vi "Generate RPC Messages.vi"(6 "Enum Metadata":T4[](array[typedef]), 7 "Messages Metadata":T5[](array[typedef]), 8 "error in (no error)":errorcluster, 11 "Library":refnum<vi>) -> (0 "error out":errorcluster, 3 "Library":refnum<vi>)   [LabVIEW 2019, in "gRPC Template Creation Utility.lvlib"]
uses:
  gRPC Template Creation Utility.lvlib
  TypeDefs/Message Metadata (Scripting).ctl
  TypeDefs/Message Element Metadata (Scripting).ctl
  TypeDefs/Message Element Type.ctl
  TypeDefs/Enum Metadata (Scripting).ctl
  TypeDefs/Oneof Metadata.ctl
panel:
  in  "Oneof Metadata":T1[](array[typedef])
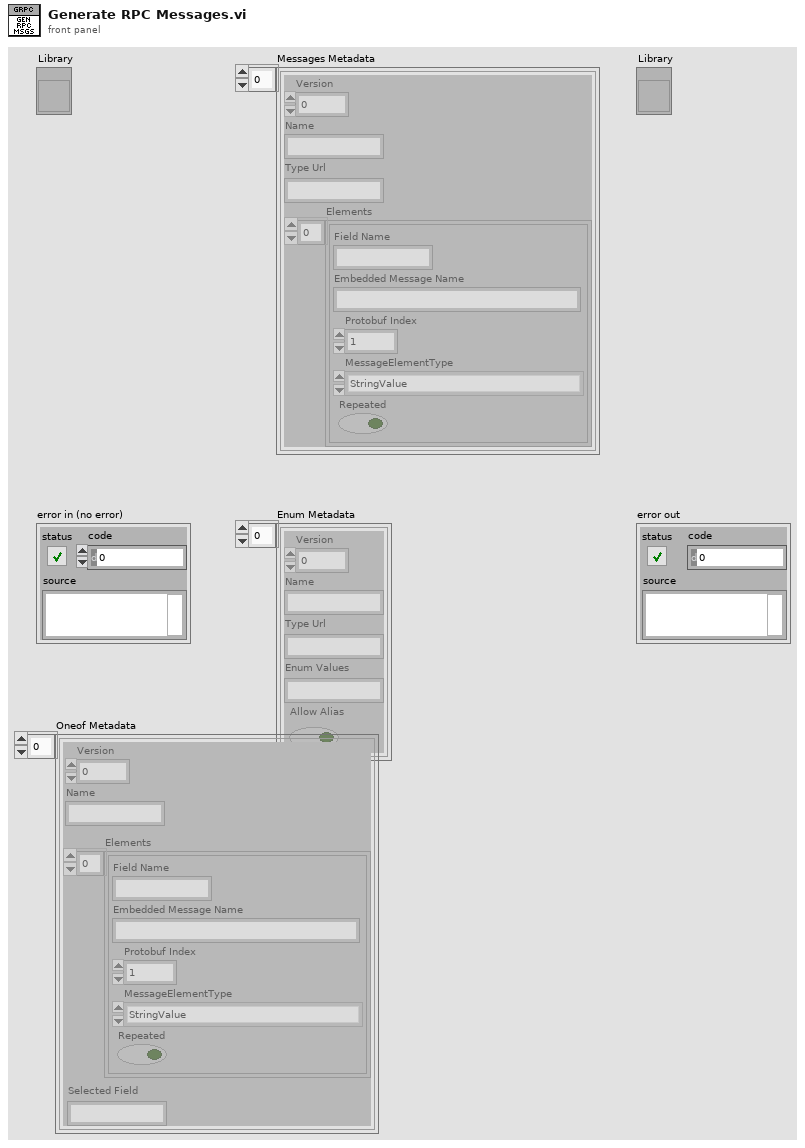
[diagram p1: front panel]
types:
  T1 = typedef "gRPC Template Creation Utility.lvlib/Oneof Metadata.ctl" = cluster{"Version":i32, "Name":string, "Elements":T2[], "Selected Field":string}
  T2 = typedef "gRPC Template Creation Utility.lvlib/Message Element Metadata (Scripting).ctl" = cluster{"Field Name":string, "Embedded Message Name":string, "Protobuf Index":i32, "MessageElementType":T3, "Repeated":bool}
  T3 = typedef "gRPC Template Creation Utility.lvlib/Message Element Type.ctl" = enum32{"Int32Value", "FloatValue", "DoubleValue", "BoolValue", "StringValue", "MessageValue", "Int64Value", "UInt32Value", "UInt64Value", "EnumValue", "Bytes", "Fixed64", "Fixed32", "SFixed64", "SFixed32", "SInt64", "SInt32", "Oneof"}
  T4 = typedef "gRPC Template Creation Utility.lvlib/Enum Metadata (Scripting).ctl" = cluster{"Version":i32, "Name":string, "Type Url":string, "Enum Values":string, "Allow Alias":bool}
  T5 = typedef "gRPC Template Creation Utility.lvlib/Message Metadata (Scripting).ctl" = cluster{"Version":i32, "Name":string, "Type Url":string, "Elements":T2[]}
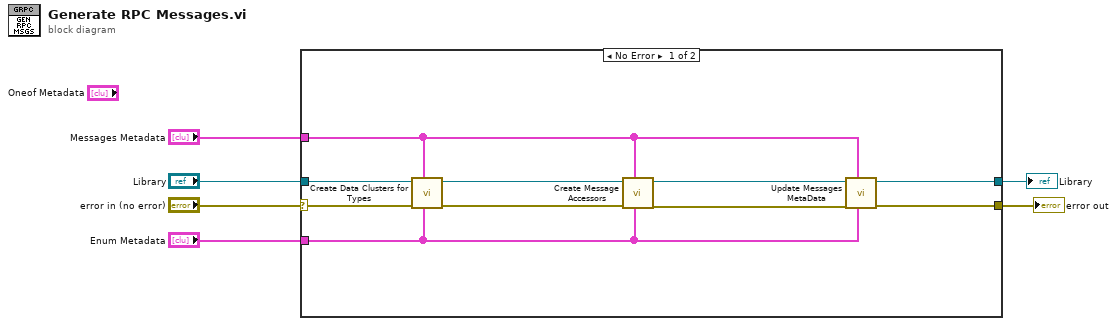
[diagram p0: block diagram]
diagram:
  n1 = case shown="No Error" "error in (no error)" {
    selector: "error in (no error)" -> [w14 w18]
    tunnel: [w13 w18] -> w6
    tunnel: [w9 w17] -> w5
    tunnel: "Messages Metadata" -> [w8 _]
    tunnel: "Library" -> [w12 w17]
    tunnel: "Enum Metadata" -> [w7 _]
    frame No Error {
      n2 = call "Create Data Clusters for Types.vi"("Enum parameters"=w7, "Message parameters"=w8, "error in (no error)"=w14, "Library in"=w12) -> ("error out"=w15:errorcluster, "Library out"=w16:refnum<vi>)  [unwired: 6 in]
      n3 = call "Create Message Accessors.vi"("Enum Parameters"=w7, "Message parameters"=w8, "error in (no error)"=w15, "Library"=w16) -> ("error out"=w11:errorcluster, "Library"=w10:refnum<vi>)  [unwired: 6 in]
      n4 = call "Update Messages MetaData.vi"("Enum MetaData"=w7, "Messages MetaData"=w8, "error in (no error)"=w11, "Library"=w10) -> ("error out"=w13:errorcluster, "Library"=w9:refnum<vi>)  [unwired: 6 in]
    }
    frame Error {
    }
  }
  "error out" <- w6
  "Library" <- w5
